vi "Open.vi"(8 "Error In":errorcluster, 10 "Enable Gestures? (T)":bool=TRUE) -> (0 "Error Out":errorcluster, 3 "Leap Handle":T1)   [LabVIEW 2011, in "LMH-Leap.lvlib"]
doc: "Leap Open allows you to open a connection to the Leap Motion Controller with the option of having gestures enabled. When <b>Enable Gestures?</b> is true, all available gestures are turned on including Circle, Swipe, Screen Tap, and Key Tap detection.\n\nIf gestures are not being used then set <b>Enable Gestures?</b> to false to reduce the amount of resource utilization required by the Leap Motion for processing gestures."
uses:
  LMH-Leap.lvlib
  Private/Type Defs/Leap Handle.ctl
  C:/github/makerhub/Leap/LabVIEW/vi.lib/MakerHub/Leap/Private/Libs/LeapCSharp.NET3.5.dll
  Private/Libs/LeapCSharp.NET3.5.dll
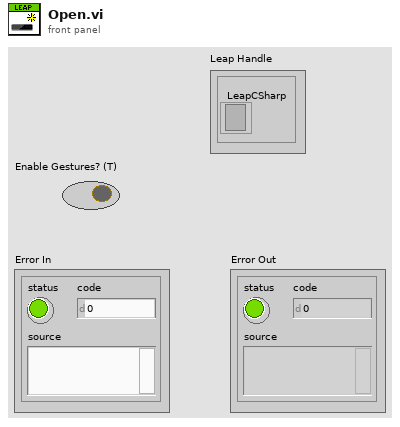
[diagram p1: front panel]
types:
  T1 = typedef "LMH-Leap.lvlib/Leap Handle.ctl" = cluster{"LeapCSharp":refnum<k24>}
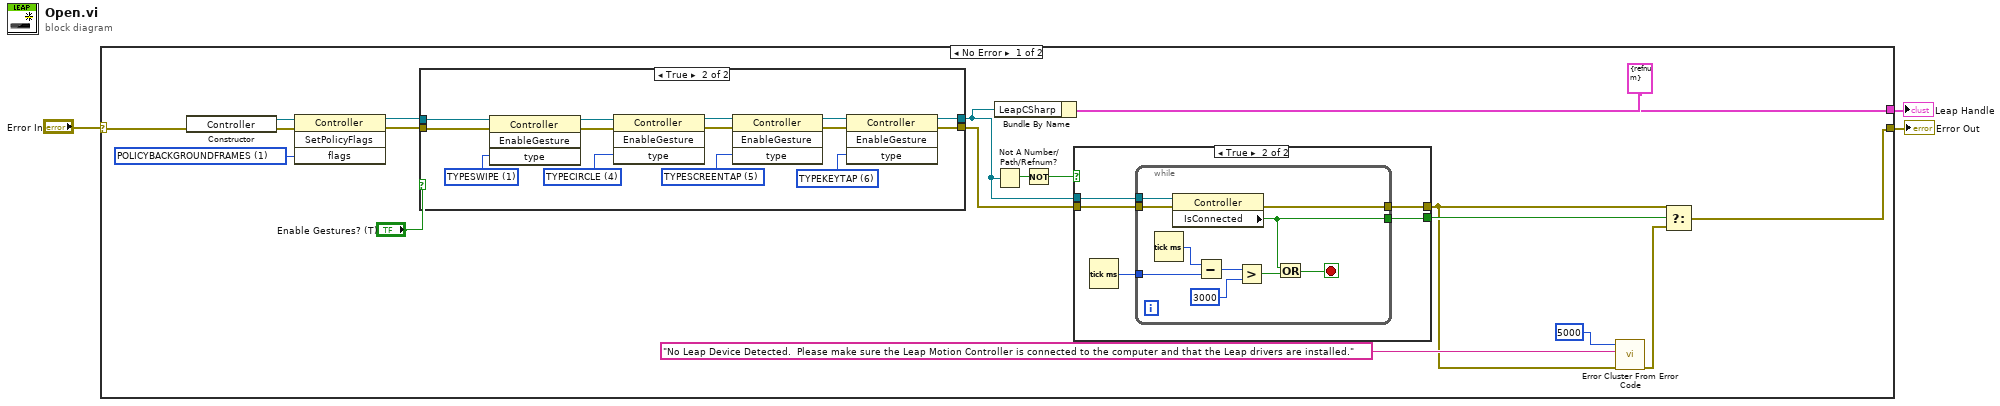
[diagram p0: block diagram]
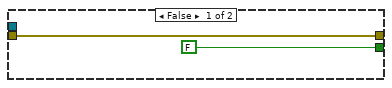
[diagram p2: hidden frame]
diagram:
  n1 = case shown="No Error" "Error In" {
    selector: "Error In" -> [w22 w56]
    tunnel: [w5 w56] -> w1
    tunnel: [w20 _] -> w3
    frame No Error {
      w14 = 1 items=["POLICYDEFAULT", "POLICYBACKGROUNDFRAMES"] ("flags")
      n2 = constructor class="Controller"(error in=w22) -> (reference out=w15:refnum<k24>, error out=w18:errorcluster)  [unwired: 2 in, 1 out]
      n3 = invoke class="Controller" method="SetPolicyFlags"(reference=w15, error in=w18, "flags"=w14) -> (reference out=w16:refnum<k24>, error out=w17:errorcluster)  [unwired: 1 in, 2 out]
      n4 = case shown="True" "Enable Gestures? (T)" {
        tunnel: w16 -> [w40 w55]
        tunnel: w17 -> [w41 w54]
        tunnel: [w41 w53] -> w10
        tunnel: [w40 w52] -> w11
        frame False {
        }
        frame True {
          w44 = 6 items=["TYPESWIPE"=1, "TYPECIRCLE"=4, "TYPESCREENTAP"=5, "TYPEKEYTAP"=6, "TYPEINVALID"=-1] ("type")
          w47 = 5 items=["TYPESWIPE"=1, "TYPECIRCLE"=4, "TYPESCREENTAP"=5, "TYPEKEYTAP"=6, "TYPEINVALID"=-1] ("type")
          w48 = 4 items=["TYPESWIPE"=1, "TYPECIRCLE"=4, "TYPESCREENTAP"=5, "TYPEKEYTAP"=6, "TYPEINVALID"=-1] ("type")
          w51 = 1 items=["TYPESWIPE"=1, "TYPECIRCLE"=4, "TYPESCREENTAP"=5, "TYPEKEYTAP"=6, "TYPEINVALID"=-1] ("type")
          n5 = invoke class="Controller" method="EnableGesture"(reference=w55, error in=w54, "type"=w51) -> (reference out=w50:refnum<k24>, error out=w49:errorcluster)  [unwired: 1 in, 2 out]
          n6 = invoke class="Controller" method="EnableGesture"(reference=w50, error in=w49, "type"=w48) -> (reference out=w46:refnum<k24>, error out=w45:errorcluster)  [unwired: 1 in, 2 out]
          n7 = invoke class="Controller" method="EnableGesture"(reference=w46, error in=w45, "type"=w47) -> (reference out=w42:refnum<k24>, error out=w43:errorcluster)  [unwired: 1 in, 2 out]
          n8 = invoke class="Controller" method="EnableGesture"(reference=w42, error in=w43, "type"=w44) -> (reference out=w52:refnum<k24>, error out=w53:errorcluster)  [unwired: 1 in, 2 out]
        }
      }
      n9 = Bundle By Name(cluster=T1 {"LeapCSharp"=refnum} ("LeapController"), "LeapCSharp"=w11) -> (w20:T1)
      n10 = Not A Number/Path/Refnum?(number/path/refnum=w11) -> (NaN/Path/Refnum?=w13:bool)
      n11 = Not(x=w13) -> (.not. x?=w12:bool)
      n12 = case shown="True" w12 {
        tunnel: w11 -> [_ w29]
        tunnel: w10 -> [w23 w28]
        tunnel: [FALSE ("IsConnected") w27] -> w9
        tunnel: [w23 w26] -> w4
        frame False {
        }
        frame True {
          n13 = Tick Count (ms)() -> (millisecond timer value=w25:u32)
          n14 = while {
            tunnel: w29 -> [w39]
            tunnel: w28 -> [w38]
            tunnel: [w31] -> w27
            tunnel: [w37] -> w26
            tunnel: w25 -> [w35]
            stop <- w30 stop-if-true
            n15 = Tick Count (ms)() -> (millisecond timer value=w36:u32)
            n16 = property class="Controller"(reference=w39, error in=w38) -> (error out=w37:errorcluster, "IsConnected"=w31:bool)  [unwired: 1 out]
            n17 = Subtract(x=w36, y=w35) -> (x-y=w34:u32)
            n18 = Greater?(x=w34, y=u32 3000) -> (0:w32:bool)
            n19 = Or(x=w31, y=w32) -> (x .or. y?=w30:bool)
          }
        }
      }
      n20 = call <vilib>:"Error Cluster From Error Code.vi"("error in (no error)"=w4, "error message (\"\")"="No Leap Device Detected.  Please make sure the Leap Motion Controller is connected to the computer and that the Leap drivers are installed." ("error message (\"\")"), "error code (0)"=5000) -> ("error out"=w6:errorcluster)  [unwired: 6 in]
      n21 = Select(t=w4, s=w9, f=w6) -> (s? t:f=w5:errorcluster)
    }
    frame Error {
    }
  }
  "Leap Handle" <- w3
  "Error Out" <- w1
